vi "State Logic.vi"(9 "Fan B Fault":bool, 10 "Fan A Fault":bool, 11 "Dual Fan in":refnum<class "Dual Fan.lvclass">) -> (0 "State Changed":bool, 1 "Fan B State":bool, 2 "Fan A State":bool, 3 "Dual Fan out":refnum<class "Dual Fan.lvclass">)   [LabVIEW 2015, in "Dual Fan.lvlib" / "Dual Fan.lvclass"]
uses:
  Dual Fan.lvclass
  Dual Fan.lvclass/Dual Fan.ctl
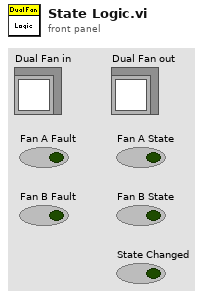
[diagram p1: front panel]
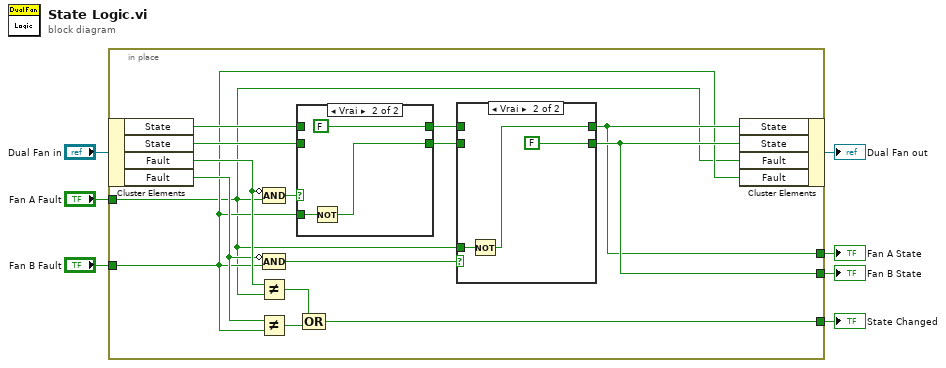
[diagram p0: block diagram]
diagram:
  n1 = in-place {
    in-place-border: [w22] -> w5
    in-place-border: [w11] -> w3
    in-place-border: [w10] -> w4
    in-place-border: "Fan B Fault" -> [w9]
    in-place-border: "Fan A Fault" -> [w8]
    n2 = in-place-cluster #1("Dual Fan in") -> ("State"=w15:bool, "State"=w14:bool, "Fault"=w13:bool, "Fault"=w12:bool)
    n3 = Not Equal?(x=w13, y=w8) -> (x != y?=w21:bool)
    n4 = Not Equal?(x=w12, y=w9) -> (x != y?=w20:bool)
    n5 = Compound Arithmetic op=AND(invert w13, w8) -> (w16:bool)
    n6 = Compound Arithmetic op=AND(invert w12, w9) -> (w17:bool)
    n7 = case shown="Vrai" w16 {
      tunnel: w9 -> [_ w32]
      tunnel: [w29 FALSE ("Fan A State")] -> w18
      tunnel: w15 -> [w29 _]
      tunnel: [w28 w30] -> w19
      tunnel: w14 -> [w28 _]
      frame False {
      }
      frame True {
        n8 = Not(x=w32) -> (.not. x?=w30:bool)
      }
    }
    n9 = Compound Arithmetic op=OR(w21, w20) -> (w22:bool)
    n10 = case shown="Vrai" w17 {
      tunnel: w8 -> [_ w27]
      tunnel: w18 -> [w24 _]
      tunnel: w19 -> [w23 _]
      tunnel: [w24 w26] -> w10
      tunnel: [w23 FALSE ("Fan A State")] -> w11
      frame False {
      }
      frame True {
        n11 = Not(x=w27) -> (.not. x?=w26:bool)
      }
    }
    n12 = in-place-cluster #1("State"=w10, "State"=w11, "Fault"=w8, "Fault"=w9) -> (→"Dual Fan out":refnum<class "Dual Fan.lvclass">)
  }
  "State Changed" <- w5
  "Fan A State" <- w4
  "Fan B State" <- w3
